vi "read output file string.vi"(8 "error in":errorcluster, 11 "shared memory editor node":refnum<class "module editor node.lvclass">) -> (0 "error out":errorcluster, 2 "output file string":string, 3 "shared memory editor node out":refnum<class "module editor node.lvclass">)   [LabVIEW 2013, in "Shared Memory editor node.lvclass"]
uses:
  Shared Memory editor node.lvclass
  <vilib>/NI/DCAF/Tag Editor Core/Configuration Editor/Classes/Module editor node/module editor node.lvclass
  module/configuration/Shared Memory configuration.lvclass
  module/configuration/Shared Memory configuration.lvclass/Shared Memory configuration.ctl
  module/configuration/Read Output File String.vi
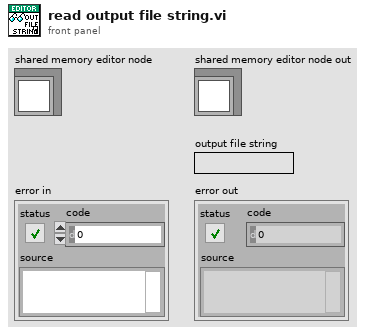
[diagram p1: front panel]
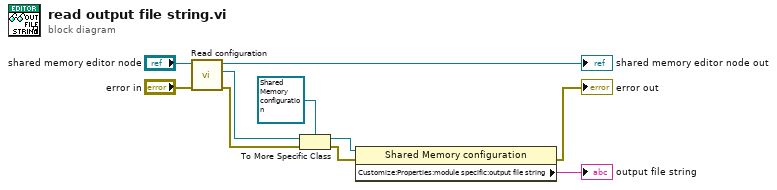
[diagram p0: block diagram]
diagram:
  n1 = call-dynamic "Read configuration.vi"("error in"="error in", "NISE_CEF_serializable node in"="shared memory editor node") -> ("error out"=w7:errorcluster, "configuration"=w8:refnum<class "NISE_CEF_serializable configuration.lvclass">, "NISE_CEF_serializable node out"=→"shared memory editor node out":refnum<class "module editor node.lvclass">)  [unwired: 7 in]
  n2 = To More Specific Class(target class=refnum<class "Shared Memory configuration.lvclass"> refnum ("shared memory configuration"), reference=w8, error in=w7) -> (specific class reference=w6:refnum<class "Shared Memory configuration.lvclass">, error out=w5:errorcluster)
  n3 = property class="Shared Memory configuration"(reference=w6, error in=w5) -> (error out=→"error out":errorcluster, "Customize:Properties:module specific:output file string"=→"output file string":string)  [unwired: 1 out]
